vi "Agg clstr mis inverter.vi"(10 "UI Refs":T1, 11 "output cluster":T2) -> ()   [LabVIEW 2019]
uses:
  controls/Parametri inverter letti.ctl
  controls/UI Data.ctl
  controls/MIS_APLUS.ctl
  DCREG/Parametri DCREG letti.ctl
  controls/Surge soglie.ctl
panel:
  # "V"
  # "[A]"
  # "[V]"
  # "[A]"
  # "[V]"
  # "V"
  # "V"
  # "[V]"
  # "[Hz]"
  # "[V]"
  # "[Hz]"
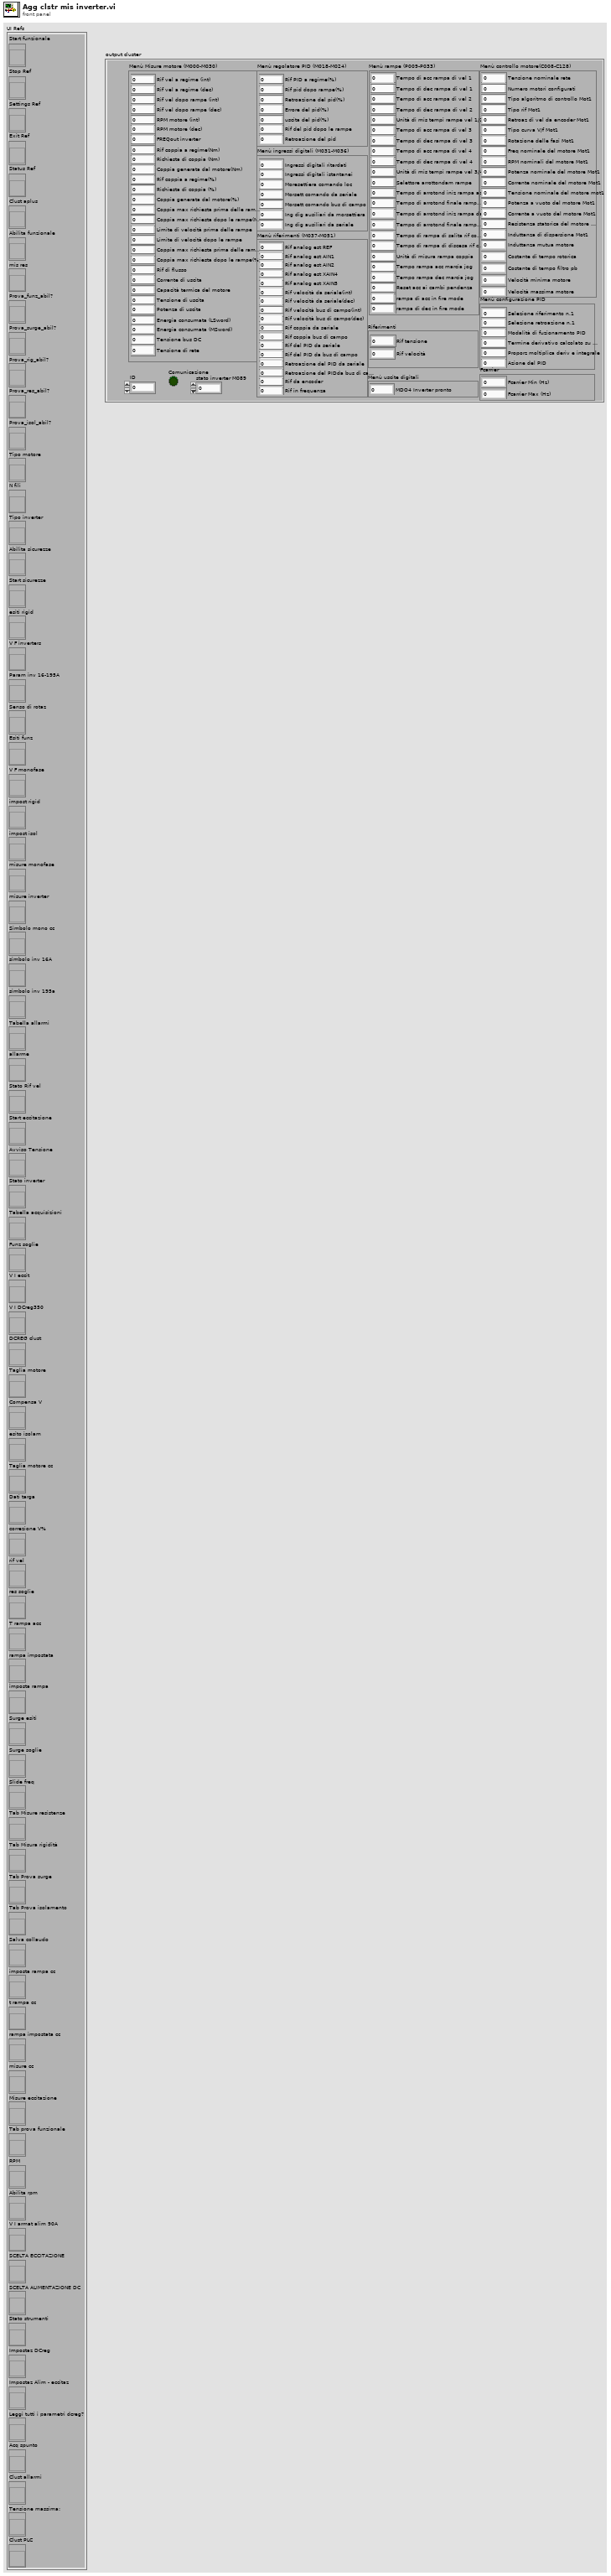
[diagram p1: front panel]
types:
  T1 = typedef "UI Data.ctl" = cluster{"Start funzionale":refnum<vi>, "Stop Ref":refnum<vi>, "Settings Ref":refnum<vi>, "Exit Ref":refnum<vi>, "Status Ref":refnum<vi>, "Clust aplus":refnum<vi>, "Abilita funzionale":refnum<vi>, "mis res":refnum<vi>, "Prova_funz_abil?":refnum<vi>, "Prova_surge_abil?":refnum<vi>, "Prova_rig_abil?":refnum<vi>, "Prova_res_abil?":refnum<vi>, "Prova_isol_abil?":refnum<vi>, "Tipo motore":refnum<vi>, "N fili":refnum<vi>, "Tipo inverter":refnum<vi>, "Abilita sicurezze":refnum<vi>, "Start sicurezze":refnum<vi>, "esiti rigid":refnum<vi>, "V F inverters":refnum<vi>, "Param inv 16-195A":refnum<vi>, "Senso di rotaz":refnum<vi>, "Esiti funz":refnum<vi>, "V F monofase":refnum<vi>, "impost rigid":refnum<vi>, "impost isol":refnum<vi>, "misure monofase":refnum<vi>, "misure inverter":refnum<vi>, "Simbolo mono cc":refnum<vi>, "simbolo inv 16A":refnum<vi>, "simbolo inv 195a":refnum<vi>, "Tabella allarmi":refnum<vi>, "allarme":refnum<vi>, "Stato Rif vel":refnum<vi>, "Start eccitazione":refnum<vi>, "Avviso Tensione":refnum<vi>, "Stato inverter":refnum<vi>, "Tabella acquisizioni":refnum<vi>, "Funz soglie":refnum<vi>, "V I eccit":refnum<vi>, "V I DCreg350":refnum<vi>, "DCREG clust":refnum<vi>, "Taglia motore":refnum<vi>, "Compensa V":refnum<vi>, "esito isolam":refnum<vi>, "Taglia motore cc":refnum<vi>, "Dati targa":refnum<vi>, "correzione V%":refnum<vi>, "rif vel":refnum<vi>, "res soglie":refnum<vi>, "T rampa acc":refnum<vi>, "rampa impostata":refnum<vi>, "imposta rampa":refnum<vi>, "Surge esiti":refnum<vi>, "Surge soglie":refnum<vi>, "Slide freq":refnum<vi>, "Tab Misure resistenze":refnum<vi>, "Tab Misura rigidità":refnum<vi>, "Tab Prova surge":refnum<vi>, "Tab Prova isolamento":refnum<vi>, "Salva collaudo":refnum<vi>, "imposta rampa cc":refnum<vi>, "t rampa cc":refnum<vi>, "rampa impostata cc":refnum<vi>, "misure cc":refnum<vi>, "Misure eccitazione":refnum<vi>, "Tab prova funzionale":refnum<vi>, "RPM":refnum<vi>, "Abilita rpm":refnum<vi>, "V I armat alim 90A":refnum<vi>, "SCELTA ECCITAZIONE":refnum<vi>, "SCELTA ALIMENTAZIONE DC":refnum<vi>, "Stato strumenti":refnum<vi>, "Impostaz DCreg":refnum<vi>, "Impostaz Alim - eccitaz":refnum<vi>, "Leggi tutti i parametri dcreg?":refnum<vi>, "Acq spunto":refnum<vi>, "Clust allarmi":refnum<vi>, "Tensione massima:":refnum<vi>, "Clust PLC":refnum<vi>}
  T2 = typedef "Parametri inverter letti.ctl" = cluster{"Menù Misure motore (M000-M030)":cluster{"Rif vel a regime (int)":u16, "Rif vel a regime (dec)":u16, "Rif vel dopo rampe (int)":u16, "Rif vel dopo rampe (dec)":u16, "RPM motore (int)":u16, "RPM motore (dec)":u16, "FREQout inverter":u16, "Rif coppia a regime(Nm)":u16, "Richiesta di coppia (Nm)":u16, "Coppia generata dal motore(Nm)":u16, "Rif coppia a regime(%)":u16, "Richiesta di coppia (%)":u16, "Coppia generata dal motore(%)":u16, "Coppia max richiesta prima delle rampe(Nm)":u16, "Coppia max richiesta dopo le rampe(Nm)":u16, "Limite di velocità prima delle rampe":u16, "Limite di velocità dopo le rampe":u16, "Coppia max richiesta prima delle rampe(%)":u16, "Coppia max richiesta dopo le rampe(%)":u16, "Rif di flusso":u16, "Corrente di uscita":u16, "Capacità termica del motore":u16, "Tensione di uscita":u16, "Potenza di uscita":u16, "Energia consumata (LSword)":u16, "Energia consumata (MSword)":u16, "Tensione bus DC":u16, "Tensione di rete":u16}, "Menù regolatore PID (M018-M024)":cluster{"Rif PID a regime(%)":u16, "Rif pid dopo rampe(%)":u16, "Retroazione del pid(%)":u16, "Errore del pid(%)":u16, "uscita del pid(%)":u16, "Rif del pid dopo le rampe":u16, "Retroazione del pid":u16}, "Menù ingressi digitali (M031-M036)":cluster{"Ingressi digitali ritardati":u16, "Ingressi digitali istantanei":u16, "Moresettiera comando loc":u16, "Morsett comando da seriale":u16, "Morsett comando bus di campo":u16, "Ing dig ausiliari da morsettiera":u16, "Ing dig ausiliari da seriale":u16}, "Menù riferimenti (M037-M051)":cluster{"Rif analog est REF":u16, "Rif analog est AIN1":u16, "Rif analog est AIN2":u16, "Rif analog est XAIN4":u16, "Rif analog est XAIN5":u16, "Rif velocità da seriale(int)":u16, "Rif velocità bus di campo(int)":u16, "Rif coppia da seriale":u16, "Rif coppia bus di campo":u16, "Rif del PID da seriale":u16, "Rif del PID da bus di campo":u16, "Retroazione del PID da seriale":u16, "Retroazione del PIDda bus di campo":u16, "Rif da encoder":u16, "Rif in frequenza":u16, "Rif velocità da seriale(dec)":u16, "Rif velocità bus di campo(dec)":u16}, "Menù rampe (P009-P033)":cluster{"Tempo di dec rampa di vel 1":u16, "Tempo di acc rampa di vel 2":u16, "Tempo di dec rampa di vel 2":u16, "Tempo di acc rampa di vel 1":u16, "Unità di mis tempi rampe vel 1/2":u16, "Tempo di acc rampa di vel 3":u16, "Tempo di dec rampa di vel 3":u16, "Tempo di acc rampa di vel 4":u16, "Tempo di dec rampa di vel 4":u16, "Unità di mis tempi rampe vel 3/4":u16, "Selettore arrottondam rampe":u16, "Tempo di arrotond iniz rampa acc":u16, "Tempo di arrotond finale rampa acc":u16, "Tempo di arrotond iniz rampa dec":u16, "Tempo di rampa di salita rif coppia":u16, "Tempo di rampa di discesa rif coppia":u16, "Unità di misura rampa coppia":u16, "Tempo rampa acc marcia jog":u16, "Tempo rampa dec marcia jog":u16, "Reset acc ai cambi pendenza":u16, "rampa di acc in fire mode":u16, "rampa di dec in fire mode":u16, "Tempo di arrotond finale rampa dec":u16}, "Menù controllo motore(C008-C128)":cluster{"Numero motori configurati":u16, "Tipo algoritmo di controllo Mot1":u16, "Tipo rif Mot1":u16, "Tensione nominale rete":u16, "Retroaz di vel da encoder Mot1":u16, "Tipo curva V/f Mot1":u16, "Rotazione delle fasi Mot1":u16, "Freq nominale del motore Mot1":u16, "RPM nominali del motore Mot1":u16, "Potenza nominale del motore Mot1":u16, "Corrente nominale del motore Mot1":u16, "Tensione nominale del motore mot1":u16, "Potenza a vuoto del motore Mot1":u16, "Corrente a vuoto del motore Mot1":u16, "Resistenza statorica del motore Mot1":u16, "Induttanza di dispersione Mot1":u16, "Induttanza mutua motore":u16, "Costante di tempo rotorica":u16, "Costante di tempo filtro pb":u16, "Velocità minima motore":u16, "Velocità massima motore":u16}, "Menù configurazione PID":cluster{"Selezione riferimento n.1":u16, "Selezione retroazione n.1":u16, "Modalità di fuzionamento PID":u16, "Termine derivativo calcolato su err o mis":u16, "Proporz moltiplica deriv e integrale":u16, "Azione del PID":u16}, "ID":dbl, "Menù uscite digitali":cluster{"MDO4 Inverter pronto":u16}, "Fcarrier":cluster{"Fcarrier Min (Hz)":u16, "Fcarrier Max (Hz)":u16}, "stato inverter M089":dbl, "Riferimenti":cluster{"Rif tensione":u16, "Rif velocità":u16}, "Comunicazione":bool}
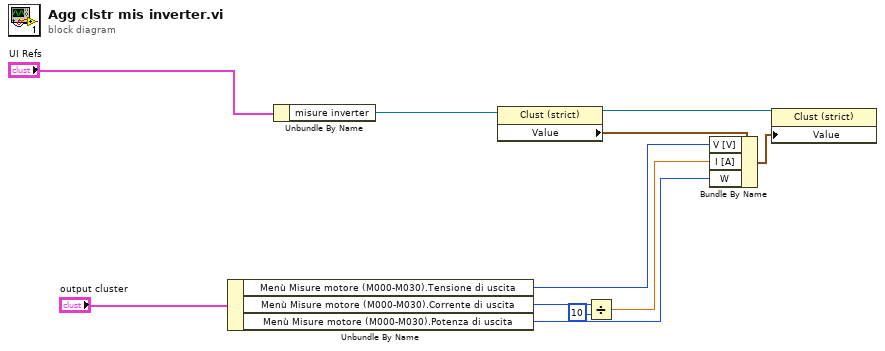
[diagram p0: block diagram]
diagram:
  n1 = Unbundle By Name("output cluster") -> ("Menù Misure motore (M000-M030).Tensione di uscita"=w9:u16, "Menù Misure motore (M000-M030).Corrente di uscita"=w7:u16, "Menù Misure motore (M000-M030).Potenza di uscita"=w11:u16)
  n2 = Unbundle By Name("UI Refs") -> ("misure inverter"=w2:refnum<vi>)
  n3 = property class="Clust (strict)"(reference=w2) -> (reference out=w4:refnum<vi>, "Value"=w3:cluster{"V [V]":dbl, "I [A]":dbl, "W":dbl})  [unwired: 1 in, 1 out]
  n4 = Divide(x=w7, y=u16 10) -> (x/y=w10:dbl)
  n5 = Bundle By Name(cluster=w3, "V [V]"=w9, "I [A]"=w10, "W"=w11) -> (w5:cluster{"V [V]":dbl, "I [A]":dbl, "W":dbl})
  n6 = property class="Clust (strict)"(reference=w4, "Value"=w5) -> ()  [unwired: 1 in, 2 out]
